vi "fast_sync_read.vi"() -> ()   [LabVIEW 2021]
uses:
  dxl_x86_c.lvlib/dxl_x86_c.lvlib
panel:
  out "dynamixel_error":string
  out "dynamixel_comm_result":string
  out "groupread_num":i32
  in  "LEN_PRESENT_POSITION":u16=4
  out "groupwrite_num":i32
  in  "LEN_GOAL_POSITION":u16=4
  out "value : PRO (knob)\npresent position 2":i32(knob) scale=150000.0..-150000.0
  in  "dynamixe2_id":u8=2
  in  "device_name":string="COM1"
  in  "ADDR_PRESENT_POSITION":u16=611
  in  "ADDR_GOAL_POSITION":u16=596
  in  "ADDR_TORQUE_ENABLE":u16=562
  out "protocol_version":dbl=2.0
  out "value : PRO (knob)\npresent position 1":i32(knob) scale=150000.0..-150000.0
  in  "terminate":bool
  out "port_num":i32
  in  "value : PRO (dial)\ngoal position":i32(knob) scale=150000.0..-150000.0
  in  "dynamixel1_id":u8=1
  in  "baud_rate":i32=57600
  # "/*******************************************************************************\n* Copyright (c) 2021, ROBOTIS CO., LTD.\n* All rights reserved.\n*\n* Redistribution and use in source and binary forms, with or without\n* modification, are permitted provided that the following conditions are met:\n*\n* * Redistributions of source code must retain the above copyright notice, this\n*   list of conditions and the following disclaimer.\n*\n* * Redistributions in binary form must reproduce the above copyright notice,\n*   this list of conditions and the following disclaimer in the documentation\n*   and/or other materials provided with the distribution.\n*\n* * Neither the name of ROBOTIS nor the names of its\n*   contributors may be used to endorse or promote products derived from\n*   this software without specific prior written permission.\n*\n* THIS SOFTWARE IS PROVIDED BY THE COPYRIGHT HOLDERS AND CONTRIBUTORS \"AS IS\"\n* AND ANY EXPRESS OR IMPLIED WARRANTIES, INCLUDING, BUT NOT LIMITED TO, THE\n* IMPLIED WARRANTIES OF MERCHANTABILITY AND FITNESS FOR A PARTICULAR PURPOSE ARE\n* DISCLAIMED. IN NO EVENT SHALL THE COPYRIGHT HOLDER OR CONTRIBUTORS BE LIABLE\n* FOR ANY DIRECT, INDIRECT, INCIDENTAL, SPECIAL, EXEMPLARY, OR CONSEQUENTIAL\n* DAMAGES (INCLUDING, BUT NOT LIMITED TO, PROCUREMENT OF SUBSTITUTE GOODS OR\n* SERVICES; LOSS OF USE, DATA, OR PROFITS; OR BUSINESS INTERRUPTION) HOWEVER\n* CAUSED AND ON ANY THEORY OF LIABILITY, WHETHER IN CONTRACT, STRICT LIABILITY,\n* OR TORT (INCLUDING NEGLIGENCE OR OTHERWISE) ARISING IN ANY WAY OUT OF THE USE\n* OF THIS SOFTWARE, EVEN IF ADVISED OF THE POSSIBILITY OF SUCH DAMAGE.\n*******************************************************************************/\n\n/* Author: Ashe kim */"
  # "Fast Sync Read Example Environment\n - Youtube : https://youtu.be/claLIK8omIQ\n\n - DYNAMIXEL: X series (except XL-320), MX(2.0) series, P series\n              ID = 1, 2, Baudrate = 57600bps, Protocol 2.0\n - USB-Serial Interface : U2D2 (DYNAMIXEL Starter Set)\n - Library: DYNAMIXEL SDK v3.8.1 or later\n\n\nAvailable Dynamixel model on this example : All models using Protocol 2.0\nThis example is designed for using a Dynamixel PRO 54-200, and an USB2DYNAMIXEL.\nTo use another Dynamixel model, such as X series, see their details in E-Manual(support.robotis.com) \n   and edit \"numeric control\"s seen left with \"Edit Text\" tool.\nBe sure that Dynamixel PRO properties are already set as %% ID : 1 / Baudnum : 1 (Baudrate : 57600)\n\n1. Run example by click above \"Run\" button (below \"Edit\" menu).\n2. Drag \"dial\" then you may see the Dynamixel and \"knob\"s rotating\n3. To finish the example, press \"terminate\" button."
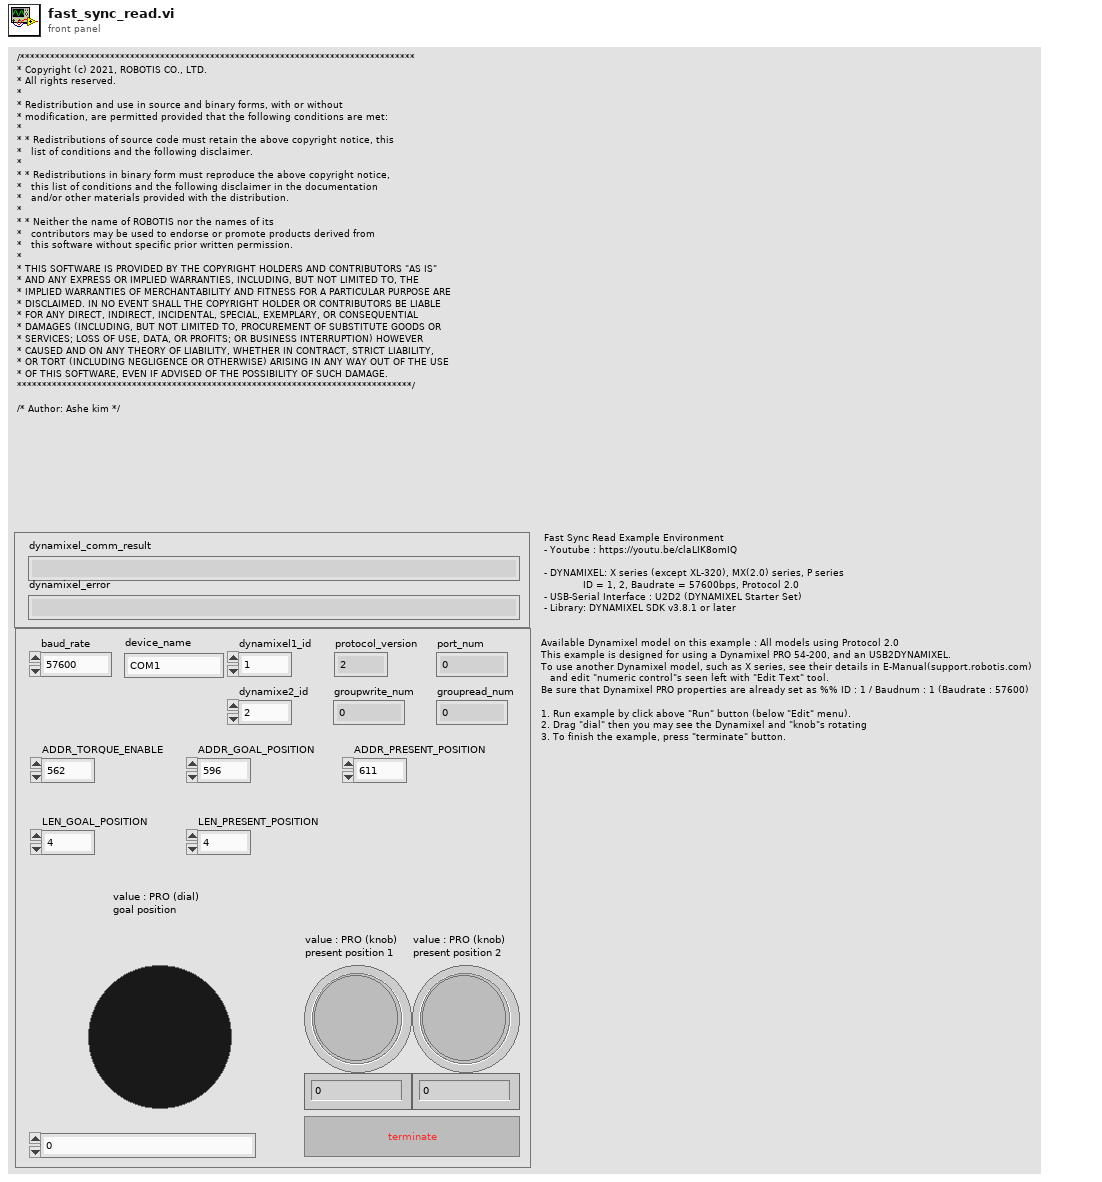
[diagram p1: front panel]
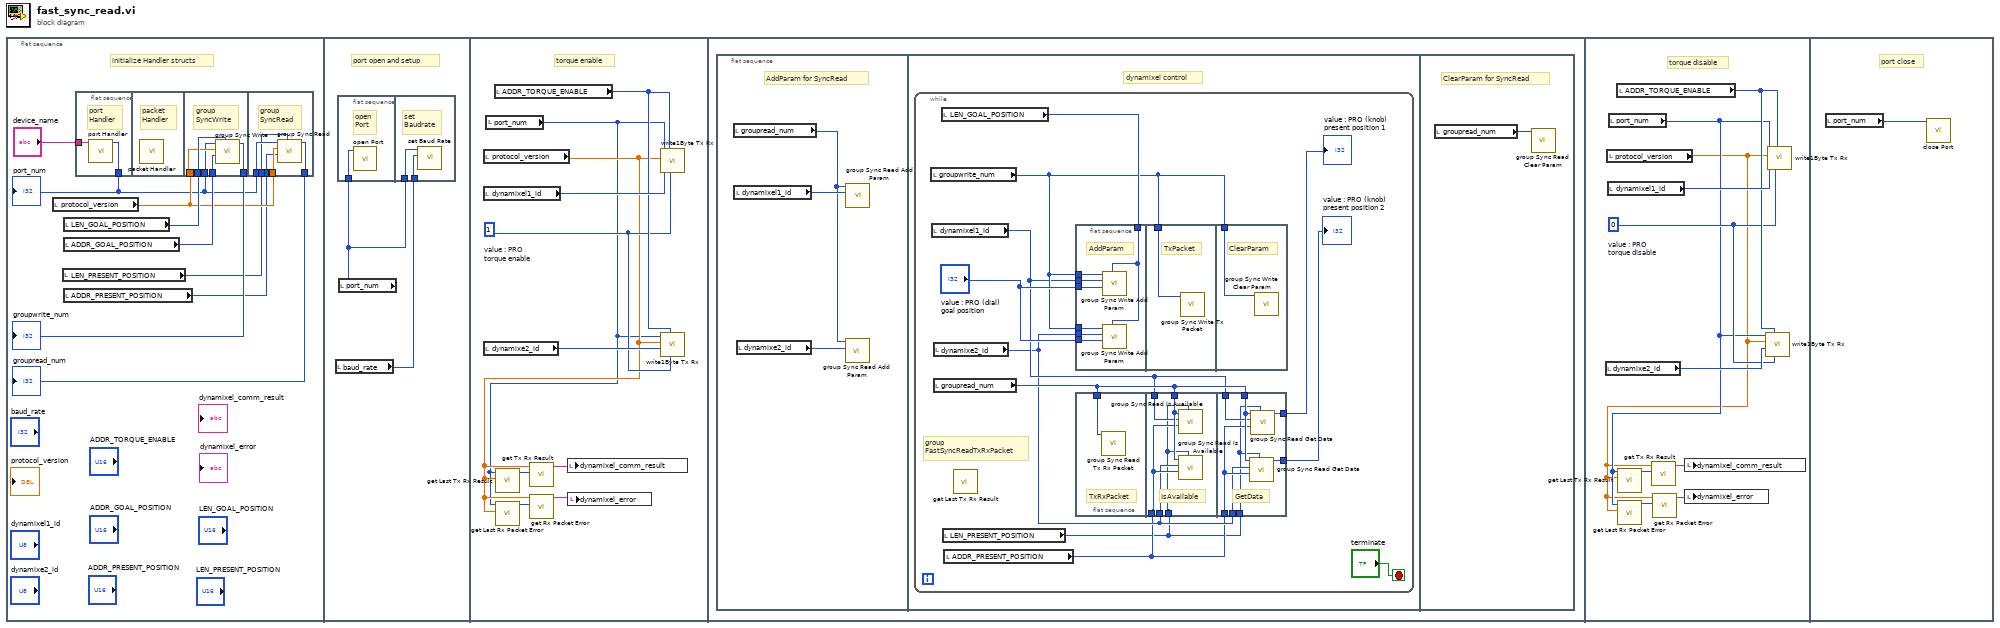
[diagram p0: block diagram]
diagram:
  n1 = flat-sequence {
    frame #0 {
      # "initialize Handler structs"
      n2 = local read "protocol_version"() -> (w4:dbl)
      n3 = local read "LEN_PRESENT_POSITION"() -> (w1:u16)
      n4 = local read "LEN_GOAL_POSITION"() -> (w8:u16)
      n5 = local read "ADDR_GOAL_POSITION"() -> (w7:u16)
      n6 = local read "ADDR_PRESENT_POSITION"() -> (w3:u16)
      n7 = flat-sequence {
        tunnel: "device_name" -> [w11]
        tunnel: [w10] -> w2
        tunnel: w8 -> [w16]
        tunnel: w7 -> [w15]
        tunnel: w4 -> [w14]
        tunnel: w2 -> [w13]
        tunnel: [w12] -> w6
        tunnel: [w21] -> w5
        tunnel: w4 -> [w20]
        tunnel: w3 -> [w19]
        tunnel: w2 -> [w18]
        tunnel: w1 -> [w17]
        frame #0 {
          # "port\nHandler"
          n8 = call "port Handler.vi"("port_name"=w11) -> ("function return"=w10:i32)  [unwired: 10 in]
        }
        frame #1 {
          # "packet\nHandler"
          n9 = call "packet Handler.vi"() -> ()  [unwired: 12 in]
        }
        frame #2 {
          # "group\nSyncWrite"
          n10 = call "group Sync Write.vi"("data_length"=w16, "start_address"=w15, "protocol_version"=w14, "port_num"=w13) -> ("function return"=w12:i32)  [unwired: 7 in]
        }
        frame #3 {
          # "group\nSyncRead"
          n11 = call "group Sync Read.vi"("data_length"=w17, "start_address"=w19, "protocol_version"=w20, "port_num"=w18) -> ("function return"=w21:i32)  [unwired: 7 in]
        }
      }
      "port_num" <- w2
      "groupwrite_num" <- w6
      "groupread_num" <- w5
    }
    frame #1 {
      # "port open and setup"
      n12 = local read "baud_rate"() -> (w22:i32)
      n13 = flat-sequence {
        tunnel: w23 -> [w24]
        tunnel: w23 -> [w26]
        tunnel: w22 -> [w25]
        frame #0 {
          # "open\nPort"
          n14 = call "open Port.vi"("port_num"=w24) -> ()  [unwired: 10 in, 1 out]
        }
        frame #1 {
          # "set\nBaudrate"
          n15 = call "set Baud Rate.vi"("baudrate"=w25, "port_num"=w26) -> ()  [unwired: 9 in, 1 out]
        }
      }
      n16 = local read "port_num"() -> (w23:i32)
    }
    frame #2 {
      w33 = 1  # value : PRO torque enable
      # "torque enable"
      n17 = local read "protocol_version"() -> (w30:dbl)
      n18 = local read "dynamixel1_id"() -> (w36:u8)
      n19 = local read "dynamixe2_id"() -> (w34:u8)
      n20 = local read "port_num"() -> (w27:i32)
      n21 = local read "ADDR_TORQUE_ENABLE"() -> (w35:u16)
      n22 = call "get Last Tx Rx Result.vi"("protocol_version"=w30, "port_num"=w27) -> ("function return"=w32:i32)  [unwired: 9 in]
      n23 = call "get Last Rx Packet Error.vi"("protocol_version"=w30, "port_num"=w27) -> ("function return"=w31:u8)  [unwired: 9 in]
      n24 = call "get Tx Rx Result.vi"("result"=w32, "protocol_version"=w30) -> ("function return"=w29:string)  [unwired: 9 in]
      n25 = call "get Rx Packet Error.vi"("error"=w31, "protocol_version"=w30) -> ("function return"=w28:string)  [unwired: 9 in]
      n26 = local write "dynamixel_comm_result"(w29) -> ()
      n27 = local write "dynamixel_error"(w28) -> ()
      n28 = call "write1Byte Tx Rx.vi"("data"=w33, "address"=w35, "id"=w36, "protocol_version"=w30, "port_num"=w27) -> ()  [unwired: 7 in]
      n29 = call "write1Byte Tx Rx.vi"("data"=w33, "address"=w35, "id"=w34, "protocol_version"=w30, "port_num"=w27) -> ()  [unwired: 7 in]
    }
    frame #3 {
      n30 = flat-sequence {
        frame #0 {
          # "AddParam for SyncRead"
          n31 = local read "groupread_num"() -> (w37:i32)
          n32 = local read "dynamixel1_id"() -> (w39:u8)
          n33 = local read "dynamixe2_id"() -> (w38:u8)
          n34 = call "group Sync Read Add Param.vi"("id"=w38, "group_num"=w37) -> ()  [unwired: 9 in, 1 out]
          n35 = call "group Sync Read Add Param.vi"("id"=w39, "group_num"=w37) -> ()  [unwired: 9 in, 1 out]
        }
        frame #1 {
          # "dynamixel control"
          n36 = while {
            stop <- "terminate" stop-if-true
            # "group\nFastSyncReadTxRxPacket"
            n37 = local read "groupwrite_num"() -> (w47:i32)
            n38 = local read "dynamixel1_id"() -> (w45:u8)
            n39 = local read "dynamixe2_id"() -> (w44:u8)
            n40 = local read "groupread_num"() -> (w46:i32)
            n41 = local read "LEN_GOAL_POSITION"() -> (w49:u16)
            n42 = local read "LEN_PRESENT_POSITION"() -> (w42:u16)
            n43 = local read "ADDR_PRESENT_POSITION"() -> (w43:u16)
            n44 = call "get Last Tx Rx Result.vi"() -> ()  [unwired: 11 in, 1 out]
            n45 = flat-sequence {
              tunnel: w49 -> [w70]
              tunnel: w47 -> [w69]
              tunnel: w47 -> [w68]
              tunnel: w45 -> [w67]
              tunnel: w44 -> [w66]
              tunnel: "value : PRO (dial)\ngoal position" -> [w65]
              tunnel: "value : PRO (dial)\ngoal position" -> [w64]
              tunnel: w47 -> [w71]
              tunnel: w47 -> [w72]
              frame #0 {
                # "AddParam"
                n46 = call "group Sync Write Add Param.vi"("data_length"=w70, "data"=w64, "id"=w67, "group_num"=w69) -> ()  [unwired: 7 in, 1 out]
                n47 = call "group Sync Write Add Param.vi"("data_length"=w70, "data"=w65, "id"=w66, "group_num"=w68) -> ()  [unwired: 7 in, 1 out]
              }
              frame #1 {
                # "TxPacket"
                n48 = call "group Sync Write Tx Packet.vi"("group_num"=w71) -> ()  [unwired: 11 in]
              }
              frame #2 {
                # "ClearParam"
                n49 = call "group Sync Write Clear Param.vi"("group_num"=w72) -> ()  [unwired: 11 in]
              }
            }
            n50 = flat-sequence {
              tunnel: w46 -> [w51]
              tunnel: w46 -> [w56]
              tunnel: w45 -> [w55]
              tunnel: w44 -> [w53]
              tunnel: w43 -> [w54]
              tunnel: w42 -> [w52]
              tunnel: w46 -> [w63]
              tunnel: w45 -> [w62]
              tunnel: w44 -> [w58]
              tunnel: w43 -> [w59]
              tunnel: w42 -> [w57]
              tunnel: [w61] -> w41
              tunnel: [w60] -> w40
              frame #0 {
                # "TxRxPacket"
                n51 = call "group Sync Read Tx Rx Packet.vi"("group_num"=w51) -> ()  [unwired: 11 in]
              }
              frame #1 {
                # "IsAvailable"
                n52 = call "group Sync Read Is Available.vi"("data_length"=w52, "address"=w54, "id"=w55, "group_num"=w56) -> ()  [unwired: 7 in, 1 out]
                n53 = call "group Sync Read Is Available.vi"("data_length"=w52, "address"=w54, "id"=w53, "group_num"=w56) -> ()  [unwired: 7 in, 1 out]
              }
              frame #2 {
                # "GetData"
                n54 = call "group Sync Read Get Data.vi"("data_length"=w57, "address"=w59, "id"=w58, "group_num"=w63) -> ("function return"=w60:u32)  [unwired: 7 in]
                n55 = call "group Sync Read Get Data.vi"("data_length"=w57, "address"=w59, "id"=w62, "group_num"=w63) -> ("function return"=w61:u32)  [unwired: 7 in]
              }
            }
            "value : PRO (knob)\npresent position 1" <- w41
            "value : PRO (knob)\npresent position 2" <- w40
          }
        }
        frame #2 {
          # "ClearParam for SyncRead"
          n56 = local read "groupread_num"() -> (w73:i32)
          n57 = call "group Sync Read Clear Param.vi"("group_num"=w73) -> ()  [unwired: 11 in]
        }
      }
    }
    frame #4 {
      w80 = 0  # value : PRO torque disable
      # "torque disable"
      n58 = local read "dynamixe2_id"() -> (w81:u8)
      n59 = local read "protocol_version"() -> (w76:dbl)
      n60 = local read "dynamixel1_id"() -> (w83:u8)
      n61 = local read "port_num"() -> (w77:i32)
      n62 = local read "ADDR_TORQUE_ENABLE"() -> (w82:u16)
      n63 = call "get Last Tx Rx Result.vi"("protocol_version"=w76, "port_num"=w77) -> ("function return"=w78:i32)  [unwired: 9 in]
      n64 = call "get Last Rx Packet Error.vi"("protocol_version"=w76, "port_num"=w77) -> ("function return"=w79:u8)  [unwired: 9 in]
      n65 = call "get Tx Rx Result.vi"("result"=w78, "protocol_version"=w76) -> ("function return"=w75:string)  [unwired: 9 in]
      n66 = call "get Rx Packet Error.vi"("error"=w79, "protocol_version"=w76) -> ("function return"=w74:string)  [unwired: 9 in]
      n67 = local write "dynamixel_comm_result"(w75) -> ()
      n68 = local write "dynamixel_error"(w74) -> ()
      n69 = call "write1Byte Tx Rx.vi"("data"=w80, "address"=w82, "id"=w81, "protocol_version"=w76, "port_num"=w77) -> ()  [unwired: 7 in]
      n70 = call "write1Byte Tx Rx.vi"("data"=w80, "address"=w82, "id"=w83, "protocol_version"=w76, "port_num"=w77) -> ()  [unwired: 7 in]
    }
    frame #5 {
      # "port close"
      n71 = local read "port_num"() -> (w84:i32)
      n72 = call "close Port.vi"("port_num"=w84) -> ()  [unwired: 11 in]
    }
  }
